vi "create daemon exec.vi"(8 "error in (no error)":errorcluster) -> (0 "error out":errorcluster)   [LabVIEW 2016, in "数据传输系统-06.lvlib" / "update.lvlib"]
uses:
  update.lvlib
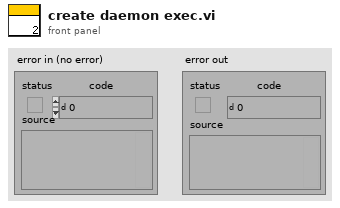
[diagram p1: front panel]
types:
  T1 = enum16{"open", "replace", "create", "open or create", "replace or create", "replace or create with confirmation"}
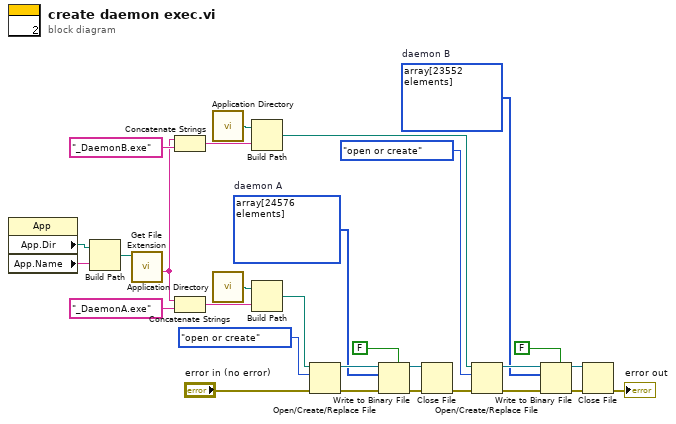
[diagram p0: block diagram]
diagram:
  w4 = u8[] array[23552 elements]  # daemon B
  w5 = u8[] array[24576 elements]  # daemon A
  n1 = property class="App"() -> ("App.Dir"=w3:path, "App.Name"=w2:string)  [unwired: 2 in, 2 out]
  n2 = Build Path(base path=w3, name or relative path=w2) -> (appended path=w1:path)
  n3 = call <vilib>:"Get File Extension.vi"("file"=w1) -> ("filename without extension"=w9:string)  [unwired: 6 in, 4 out]
  n4 = Concatenate Strings(w9, "_DaemonB.exe" ("名称或相对路径")) -> (w8:string)
  n5 = Concatenate Strings(w9, "_DaemonA.exe" ("名称或相对路径")) -> (w11:string)
  n6 = call <vilib>:"Application Directory.vi"() -> ("Application Directory"=w14:path)
  n7 = call <vilib>:"Application Directory.vi"() -> ("Application Directory"=w29:path)
  n8 = Build Path(base path=w14, name or relative path=w8) -> (appended path=w15:path)
  n9 = Build Path(base path=w29, name or relative path=w11) -> (appended path=w28:path)
  n10 = Open/Create/Replace File(file path (use dialog)=w28, error in="error in (no error)", operation (0:open)=T1."open or create" ("操作(0:open)")) -> (refnum out=w26:refnum<file>, error out=w25:errorcluster)  [unwired: 3 in, 1 out]
  n11 = Write to Binary File(file (use dialog)=w26, data=w5, error in=w25, 5:FALSE ("预置数组或字符串大小？ (T)")) -> (refnum out=w22:refnum<file>, error out=w23:errorcluster)  [unwired: 2 in, 1 out]
  n12 = Close File(refnum=w22, error in=w23) -> (error out=w13:errorcluster)  [unwired: 1 out]
  n13 = Open/Create/Replace File(file path (use dialog)=w15, error in=w13, operation (0:open)=T1."open or create" ("操作(0:open)")) -> (refnum out=w17:refnum<file>, error out=w18:errorcluster)  [unwired: 3 in, 1 out]
  n14 = Write to Binary File(file (use dialog)=w17, data=w4, error in=w18, 5:FALSE ("预置数组或字符串大小？ (T)")) -> (refnum out=w21:refnum<file>, error out=w20:errorcluster)  [unwired: 2 in, 1 out]
  n15 = Close File(refnum=w21, error in=w20) -> (error out=→"error out":errorcluster)  [unwired: 1 out]
